vi "Recieve Result.vi"(8 "error in (no error)":errorcluster, 10 "Mag Lab Result.lvclass":refnum<class "Mag Lab Result.lvclass">, 11 "Common Measurements in":refnum<class "Common Measurements.lvclass">) -> (0 "error out":errorcluster, 3 "Common Measurements out":refnum<class "Common Measurements.lvclass">)   [LabVIEW 2015, in "Common Measurements.lvclass"]
uses:
  Common Measurements.lvclass
  Mag Lab Result/Mag Lab Result.lvclass
  Compound Measurement/Compound Measurement.lvclass/Compound Measurement.ctl
  Mag Lab Root/Mag Lab Root.lvclass/Mag Lab Root.ctl
  Mag Lab Result/Mag Lab Result.lvclass/Mag Lab Result.ctl
  Mag Lab Result/Read Name.vi
  Mag Lab Result/Write Group Name.vi
  Compound Measurement/Read Results.vi
  Compound Measurement/Read Awaiting Results.vi
  Mag Lab Root/Read Synchronous operation.vi
  Mag Lab Error Handler/Mag Lab Error Handler.lvclass
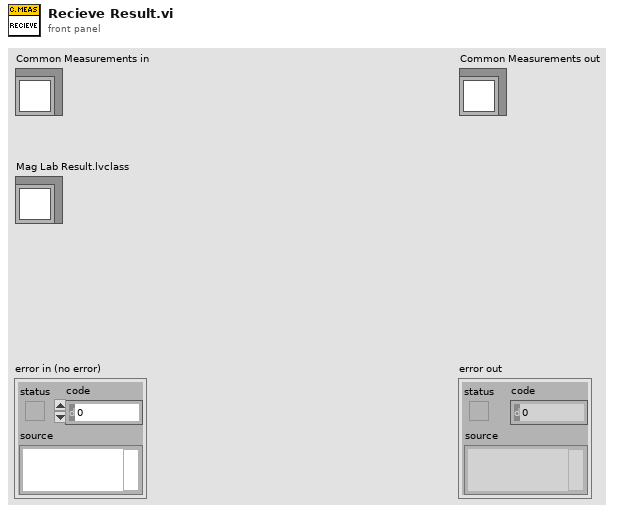
[diagram p1: front panel]
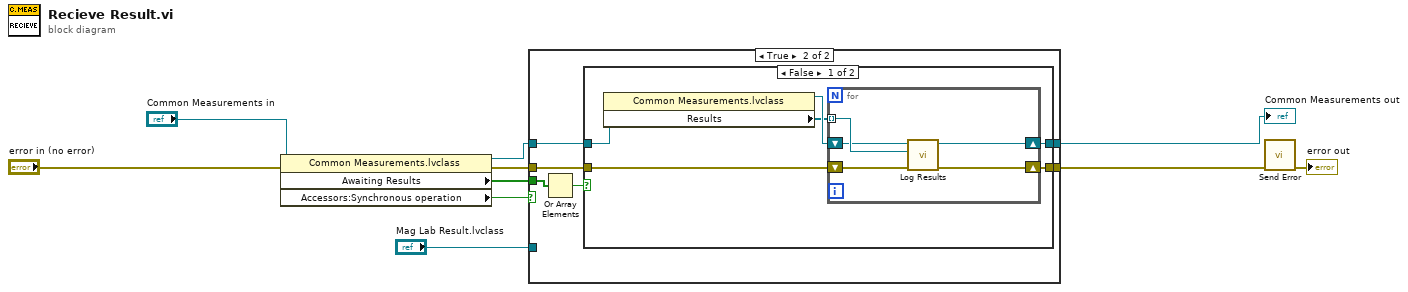
[diagram p0: block diagram]
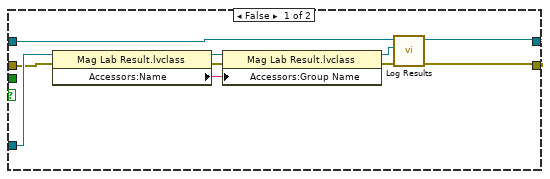
[diagram p2: hidden frame]
diagram:
  n1 = property class="Common Measurements.lvclass"(reference="Common Measurements in", error in="error in (no error)") -> (reference out=w6:refnum<class "Common Measurements.lvclass">, error out=w1:errorcluster, "Awaiting Results"=w5:bool[], "Accessors:Synchronous operation"=w4:bool)
  n2 = case shown="True" w4 {
    tunnel: [w19 w26] -> w9
    tunnel: w1 -> [w17 w25]
    tunnel: [w11 w24] -> w8
    tunnel: w6 -> [w20 w23]
    tunnel: w5 -> [_ w22]
    tunnel: "Mag Lab Result.lvclass" -> [w18 _]
    frame False {
      n3 = property class="Mag Lab Result.lvclass"(reference=w18, error in=w17) -> (reference out=w16:refnum<class "Mag Lab Result.lvclass">, error out=w15:errorcluster, "Accessors:Name"=w14:string)
      n4 = property class="Mag Lab Result.lvclass"(reference=w16, error in=w15, "Accessors:Group Name"=w14) -> (reference out=w13:refnum<class "Mag Lab Result.lvclass">, error out=w12:errorcluster)
      n5 = call-dynamic "Log Results.vi"("error in (no error)"=w12, "Result"=w13, "Common Measurements in"=w20) -> ("error out"=w11:errorcluster, "Common Measurements out"=w19:refnum<class "Common Measurements.lvclass">)  [unwired: 7 in]
    }
    frame True {
      n6 = Or Array Elements(Boolean array=w22) -> (logical OR=w21:bool)
      n7 = case shown="False" w21 {
        tunnel: [w32 w38] -> w26
        tunnel: w25 -> [w31 w39]
        tunnel: [w30 w39] -> w24
        tunnel: w23 -> [w29 w38]
        frame False {
          n8 = property class="Common Measurements.lvclass"(reference=w29) -> (reference out=w28:refnum<class "Common Measurements.lvclass">, "Results"=w27:refnum<class "Mag Lab Result.lvclass">[])  [unwired: 1 in, 1 out]
          n9 = for {
            tunnel: w27 -> [w36] mode=indexing
            shift-right: [w34] -> w30
            shift-left: w31 -> [w35]
            shift-right: [w37] -> w32
            shift-left: w28 -> [w33]
            n10 = call-dynamic "Log Results.vi"("error in (no error)"=w35, "Result"=w36, "Common Measurements in"=w33) -> ("error out"=w34:errorcluster, "Common Measurements out"=w37:refnum<class "Common Measurements.lvclass">)  [unwired: 7 in]
          }
        }
        frame True {
        }
      }
    }
  }
  "Common Measurements out" <- w9
  n11 = call "Send Error.vi"("error in (no error)"=w8) -> ("error out"=→"error out":errorcluster)  [unwired: 9 in, 1 out]
